vi "IVScaleYAxis.vi"(9 "Data IN":cluster{dbl[], dbl[], dbl[], dbl[], dbl[]}[](array[cluster]), 10 "Plot In":cluster{dbl[], dbl[]}[](graph), 11 "Y Scale":enum16{"nanoAmps", "microAmps", "milliAmps"}(ring)) -> (2 "Plot Out":cluster{dbl[], dbl[]}[](array[cluster]))   [LabVIEW 2019]
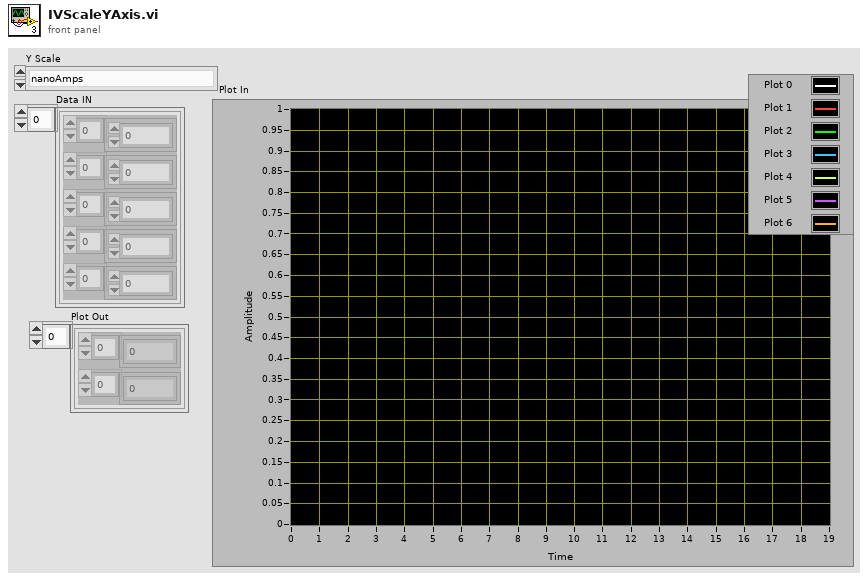
[diagram p1: front panel]
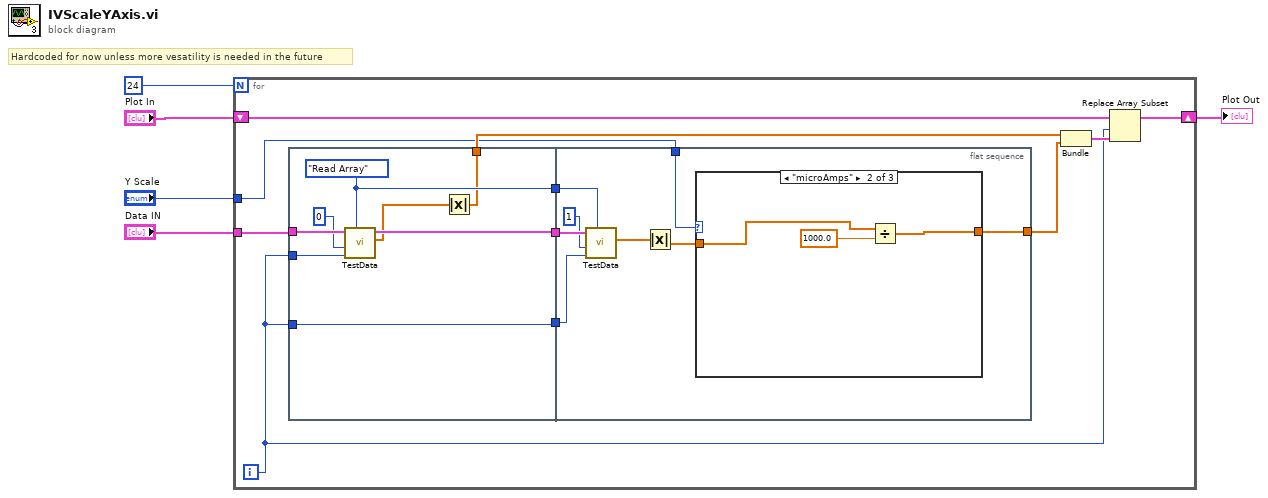
[diagram p0: block diagram]
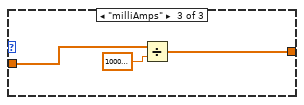
[diagram p3: hidden frame]
diagram:
  # "Hardcoded for now unless more vesatility is needed in the future"
  n1 = for {
    N: 24 -> [_]
    tunnel: "Y Scale" -> [w6]
    tunnel: "Data IN" -> [w16]
    shift-right: [w7] -> w2
    shift-left: "Plot In" -> [w8]
    i -> [w9]
    n2 = flat-sequence {
      tunnel: w16 -> [w24]
      tunnel: [w23] -> w15
      tunnel: w9 -> [w21]
      tunnel: [w19] -> w14
      tunnel: w9 -> [w19]
      tunnel: [w18] -> w13
      tunnel: [w17] -> w11
      tunnel: w15 -> [w31]
      tunnel: w14 -> [w30]
      tunnel: w13 -> [w29]
      tunnel: [w27] -> w12
      tunnel: w6 -> [w26]
      frame #0 {
        w18 = enum16{"Reset", "Write Element", "Read Array"}."Read Array" ("Action")
        n3 = call "TestData.vi"("Action"=w18, "Test No."=w21, "Array No."=u32 0, "Data IN"=w24) -> ("Array OUT"=w22:dbl[], "Data OUT"=w23:cluster{dbl[], dbl[], dbl[], dbl[], dbl[]}[])  [unwired: 6 in]
        n4 = Absolute Value(x=w22) -> (abs(x)=w17:dbl[])
      }
      frame #1 {
        n5 = call "TestData.vi"("Action"=w29, "Test No."=w30, "Array No."=u32 1, "Data IN"=w31) -> ("Array OUT"=w28:dbl[])  [unwired: 6 in, 1 out]
        n6 = Absolute Value(x=w28) -> (abs(x)=w32:dbl[])
        n7 = case shown="\"microAmps\"" w26 {
          tunnel: [w33 w34 w38] -> w27
          tunnel: w32 -> [w33 w36 w39]
          frame "nanoAmps" {
          }
          frame "microAmps" {
            n8 = Divide(x=w36, y=1000.0) -> (x/y=w34:dbl[])
          }
          frame "milliAmps" {
            n9 = Divide(x=w39, y=1000000.0) -> (x/y=w38:dbl[])
          }
        }
      }
    }
    n10 = Bundle(w11, w12) -> (w10:cluster{dbl[], dbl[]})  [unwired: 1 in]
    n11 = Replace Array Subset(array=w8, new element=w10, index=w9) -> (w7:cluster{dbl[], dbl[]}[])
  }
  "Plot Out" <- w2
